vi "Get Binary.vi"(4 "Source (\"\")":string, 8 "error in (no error)":errorcluster, 11 "VISA resource name":refnum<visa-resource-name>) -> (0 "error out":errorcluster, 1 "End of Data":bool, 2 "Binary Data":string, 3 "VISA resource name out":refnum<visa-resource-name>, 5 "Read count":i32)   [LabVIEW 2020, in "Yokogawa GX Series.lvlib"]
doc: "This VI gets Binary data.\nSend Message, then recieve the response. If Response Type is Binary, remained datas are recieved by this VI."
uses:
  <instrlib>/Yokogawa GX Series/Yokogawa GX Series.lvlib
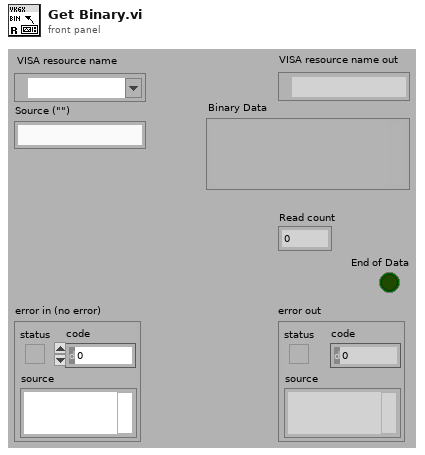
[diagram p1: front panel]
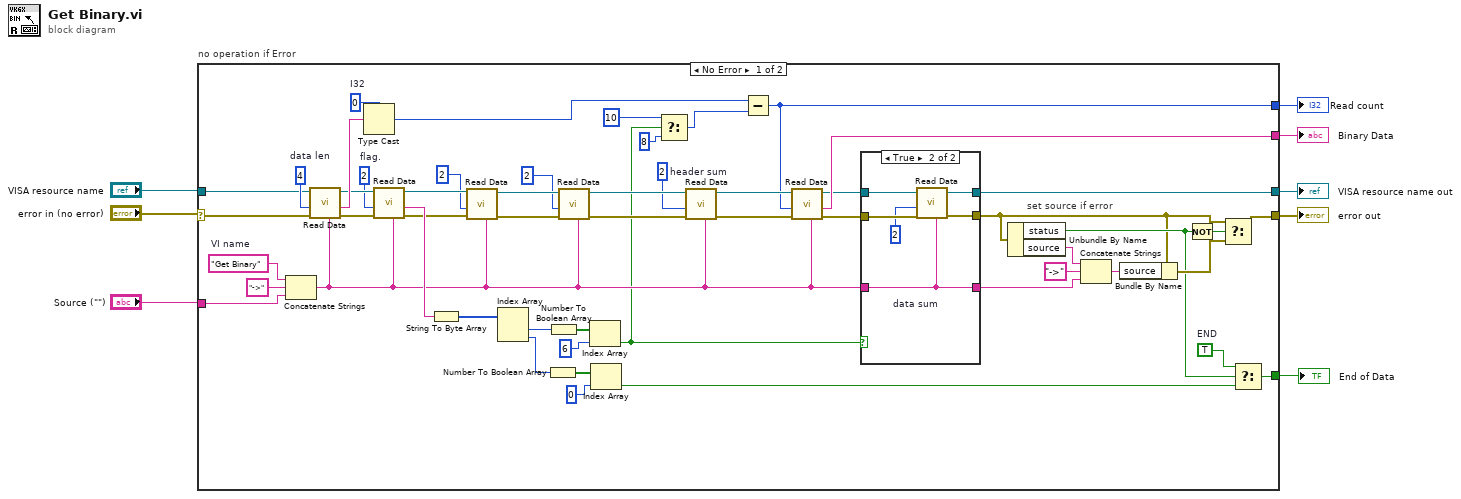
[diagram p0: block diagram]
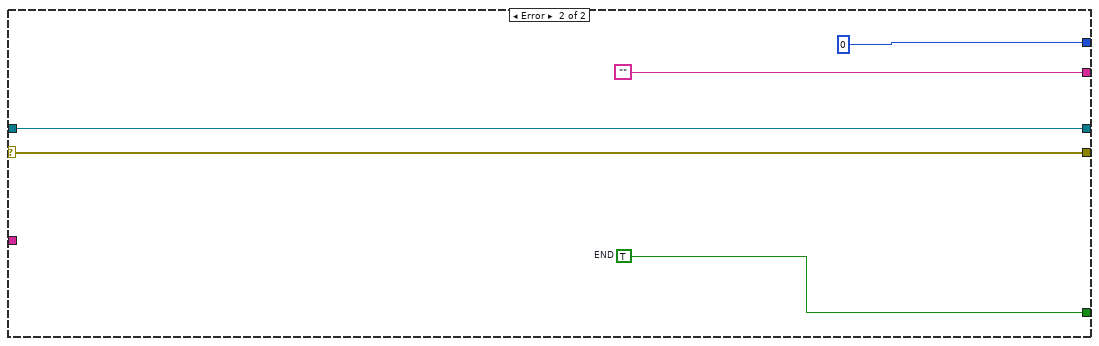
[diagram p3: hidden frame]
diagram:
  n1 = case "no operation if Error" shown="No Error" "error in (no error)" {
    selector: "error in (no error)" -> [w35 w74]
    tunnel: [w20 w72] -> w2
    tunnel: [w42 ""] -> w5
    tunnel: [w57 w74] -> w3
    tunnel: [w36 w75] -> w4
    tunnel: "VISA resource name" -> [w47 w75]
    tunnel: "Source (\"\")" -> [w31 _]
    tunnel: [w21 0] -> w1
    frame No Error {
      w13 = 2  # header sum
      w33 = "Get Binary"  # VI name
      w34 = TRUE  # END
      w48 = 4  # data len
      w43 = 2  # flag.
      w50 = 0  # I32
      # "set source if error"
      n2 = Concatenate Strings(w33, "->", w31) -> (w15:string)
      n3 = call <instrlib>:"Read Data.vi"("Source (\"\")"=w15, "error in (no error)"=w35, "Byte (0)"=w48, "VISA resource name"=w47) -> ("error out"=w45:errorcluster, "Read Buffer"=w49:string, "VISA resource name out"=w44:refnum<visa-resource-name>)  [unwired: 5 out]
      n4 = Type Cast(type=w50, x=w49) -> (*(type *) &x=w58:i32)
      n5 = call <instrlib>:"Read Data.vi"("Source (\"\")"=w15, "error in (no error)"=w45, "Byte (0)"=w43, "VISA resource name"=w44) -> ("error out"=w29:errorcluster, "Read Buffer"=w46:string, "VISA resource name out"=w30:refnum<visa-resource-name>)  [unwired: 5 out]
      n6 = String To Byte Array(string=w46) -> (unsigned byte array=w59:u8[])
      n7 = call <instrlib>:"Read Data.vi"("Source (\"\")"=w15, "error in (no error)"=w29, "Byte (0)"=2, "VISA resource name"=w30) -> ("error out"=w27:errorcluster, "VISA resource name out"=w28:refnum<visa-resource-name>)  [unwired: 6 out]
      n8 = Index Array(array=w59) -> (element #1=w18:u8, element #2=w19:u8)  [unwired: 2 in]
      n9 = Number To Boolean Array(number=w19) -> (Boolean array=w60:bool[])
      n10 = Number To Boolean Array(number=w18) -> (Boolean array=w17:bool[])
      n11 = call <instrlib>:"Read Data.vi"("Source (\"\")"=w15, "error in (no error)"=w27, "Byte (0)"=2, "VISA resource name"=w28) -> ("error out"=w25:errorcluster, "VISA resource name out"=w26:refnum<visa-resource-name>)  [unwired: 6 out]
      n12 = Index Array(array=w17, index=6) -> (element=w12:bool)
      n13 = Index Array(array=w60, index=0) -> (element=w22:bool)
      n14 = Select(t=10, s=w12, f=8) -> (s? t:f=w9:i32)
      n15 = call <instrlib>:"Read Data.vi"("Source (\"\")"=w15, "error in (no error)"=w25, "Byte (0)"=w13, "VISA resource name"=w26) -> ("error out"=w40:errorcluster, "VISA resource name out"=w41:refnum<visa-resource-name>)  [unwired: 6 out]
      n16 = Subtract(x=w58, y=w9) -> (x-y=w21:i32)
      n17 = call <instrlib>:"Read Data.vi"("Source (\"\")"=w15, "error in (no error)"=w40, "Byte (0)"=w21, "VISA resource name"=w41) -> ("error out"=w37:errorcluster, "Read Buffer"=w42:string, "VISA resource name out"=w38:refnum<visa-resource-name>)  [unwired: 5 out]
      n18 = case shown="True" w12 {
        tunnel: [w63 w70] -> w39
        tunnel: w38 -> [w64 w69]
        tunnel: w37 -> [w63 w68]
        tunnel: [w64 w67] -> w36
        tunnel: w15 -> [w62 w65]
        tunnel: [w62 w65] -> w14
        frame False {
        }
        frame True {
          w66 = 2  # data sum
          n19 = call <instrlib>:"Read Data.vi"("Source (\"\")"=w65, "error in (no error)"=w68, "Byte (0)"=w66, "VISA resource name"=w69) -> ("error out"=w70:errorcluster, "VISA resource name out"=w67:refnum<visa-resource-name>)  [unwired: 6 out]
        }
      }
      n20 = Unbundle By Name(w39) -> ("status"=w51:bool, "source"=w56:string)
      n21 = Concatenate Strings(w56, "->", w14) -> (w54:string)
      n22 = Bundle By Name(cluster=w39, "source"=w54) -> (w53:errorcluster)
      n23 = Not(x=w51) -> (.not. x?=w52:bool)
      n24 = Select(t=w39, s=w52, f=w53) -> (s? t:f=w57:errorcluster)
      n25 = Select(t=w34, s=w51, f=w22) -> (s? t:f=w20:bool)
    }
    frame Error {
      w72 = TRUE  # END
    }
  }
  "error out" <- w3
  "VISA resource name out" <- w4
  "Binary Data" <- w5
  "End of Data" <- w2
  "Read count" <- w1
